vi "calculate s.vi"(0 "Chi_A":dbl format="%_5g", 1 "Chi_B":dbl format="%_5g", 2 "Psi_A":dbl format="%_5g", 3 "Psi_B":dbl format="%_5g", 4 "W_A [raw signal]":dbl format="%_5g", 5 "W_B [raw signal]":dbl format="%_5g", 8 "Z":dbl format="%_5g", 9 "T [K]":dbl format="%_5g", 11 "P [kPa]":dbl format="%_5g", 12 "Substance (CO2/H2O)":T1) -> (16 "S":dbl)   [LabVIEW 2017, in "LicorLI7000.lvlib"]
uses:
  LicorLI7000.lvlib
  conventions/Substance.ctl
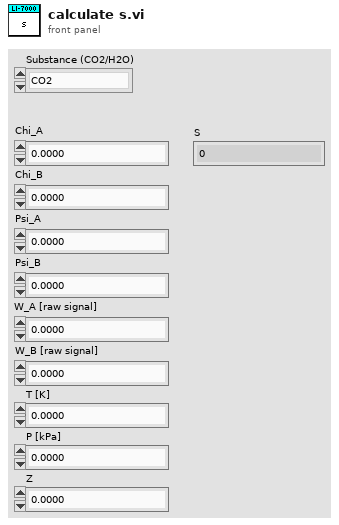
[diagram p1: front panel]
types:
  T1 = typedef "LicorLI7000.lvlib/Substance.ctl" = enum16{"CO2", "H2O"}
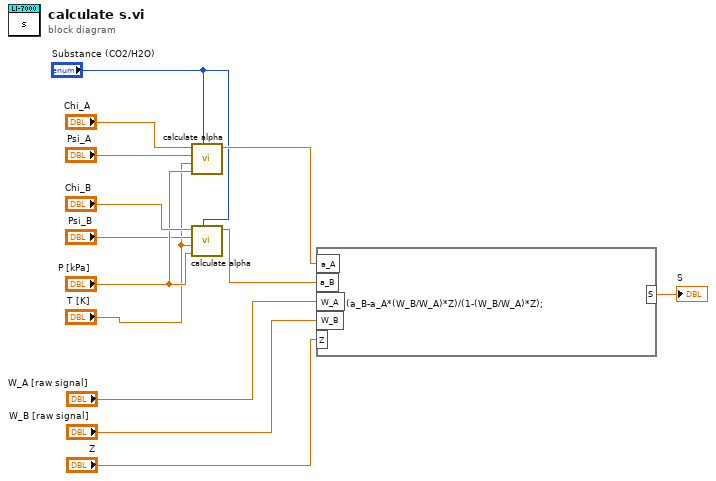
[diagram p0: block diagram]
diagram:
  n1 = call "calculate alpha.vi"("Substance (CO2/H2O)"="Substance (CO2/H2O)", "P [kPa]"="P [kPa]", "T [K]"="T [K]", "Psi_i"="Psi_A", "Chi_i"="Chi_A") -> ("absorptance_i"=w9:dbl)  [unwired: 6 in]
  n2 = call "calculate alpha.vi"("Substance (CO2/H2O)"="Substance (CO2/H2O)", "P [kPa]"="P [kPa]", "T [K]"="T [K]", "Psi_i"="Psi_B", "Chi_i"="Chi_B") -> ("absorptance_i"=w10:dbl)  [unwired: 6 in]
  n3 = formula code="S = (a_B-a_A*(W_B/W_A)*Z)/(1-(W_B/W_A)*Z);"("a_B"=w10, "a_A"=w9, "W_A"="W_A [raw signal]", "W_B"="W_B [raw signal]", "Z"="Z") -> ("S"=→"S":dbl)
